vi "ConvertToAssociationType.vi"(0 "lineStyle":T3, 1 "EndArrowHead":T2, 2 "StartArrowHead":T2) -> (14 "RelationType":T1 items=["Depenency", "Inheritance", "Interface Implementation", "Association", "Aggregation", "Composite Aggregation"], 16 "Bi sirectional":bool)   [LabVIEW 2012, in "ClassRelationshipEdge.lvclass"]
uses:
  <resource>/Framework/Providers/Open_GDS/UML/ClassRelationshipEdge_class/ClassRelationshipEdge.lvclass
  <resource>/Framework/Providers/Open_GDS/UML/ArrowHead_class/ArrowHeadType.ctl
  <resource>/Framework/Providers/Open_GDS/UML/LineStyle_class/LineStyleType.ctl
  <resource>/Framework/Providers/Open_GDS/UML/ClassRelationshipEdge_class/private/AssociationType.ctl
  <resource>/Framework/Providers/Open_GDS/UML/ArrowHead_class/ArrowHead.lvclass
  <resource>/Framework/Providers/Open_GDS/UML/LineStyle_class/LineStyle.lvclass
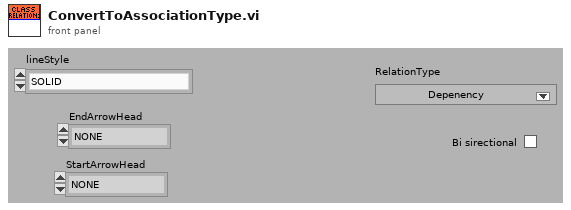
[diagram p1: front panel]
types:
  T1 = typedef "ClassRelationshipEdge.lvclass/AssociationType.ctl" = u16
  T2 = typedef "ArrowHead.lvclass/ArrowHeadType.ctl" = enum16{"NONE", "TRIANGLE", "BLACK_TRIANGLE", "V", "HALF_V", "DIAMOND", "BLACK_DIAMOND"}
  T3 = typedef "LineStyle.lvclass/LineStyleType.ctl" = enum16{"SOLID", "DOTTED"}
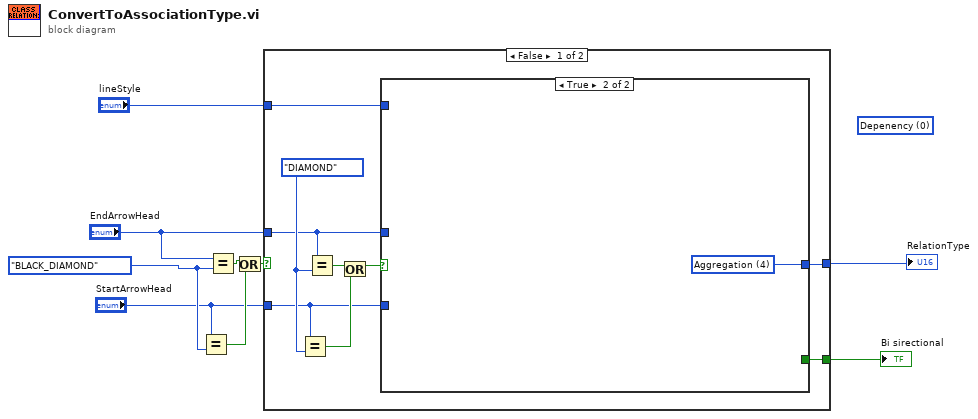
[diagram p0: block diagram]
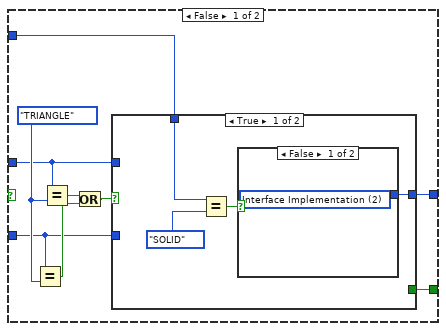
[diagram p2: hidden frame]
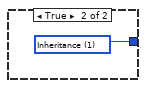
[diagram p3: hidden frame]
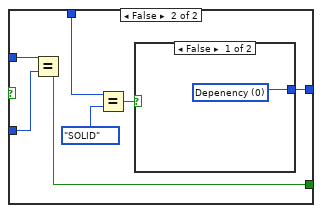
[diagram p4: hidden frame]
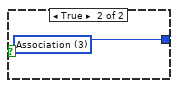
[diagram p5: hidden frame]
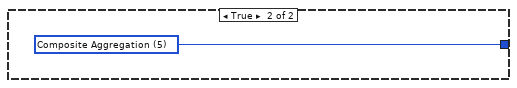
[diagram p6: hidden frame]
diagram:
  w7 = ArrowHeadType."BLACK_DIAMOND" ("y")
  (unwired) T1 0 items=["Depenency", "Inheritance", "Interface Implementation", "Association", "Aggregation", "Composite Aggregation"] ("RelationType")
  n1 = Equal?(x="StartArrowHead", y=w7) -> (x = y?=w5:bool)
  n2 = Equal?(x="EndArrowHead", y=w7) -> (x = y?=w9:bool)
  n3 = Or(x=w9, y=w5) -> (x .or. y?=w6:bool)
  n4 = case shown="False" w6 {
    tunnel: [w14 w44] -> w8
    tunnel: "StartArrowHead" -> [w12 _]
    tunnel: "EndArrowHead" -> [w13 _]
    tunnel: "lineStyle" -> [w11 _]
    tunnel: [w10 _] -> w1
    frame False {
      w16 = ArrowHeadType."DIAMOND" ("y")
      n5 = Equal?(x=w12, y=w16) -> (x = y?=w18:bool)
      n6 = Equal?(x=w13, y=w16) -> (x = y?=w17:bool)
      n7 = Or(x=w17, y=w18) -> (x .or. y?=w15:bool)
      n8 = case shown="True" w15 {
        tunnel: [w23 w43] -> w14
        tunnel: w13 -> [w21 _]
        tunnel: w12 -> [w20 _]
        tunnel: w11 -> [w22 _]
        tunnel: [w19 _] -> w10
        frame False {
          w27 = ArrowHeadType."TRIANGLE" ("y")
          n9 = Equal?(x=w20, y=w27) -> (x = y?=w25:bool)
          n10 = Equal?(x=w21, y=w27) -> (x = y?=w26:bool)
          n11 = Or(x=w26, y=w25) -> (x .or. y?=w24:bool)
          n12 = case shown="True" w24 {
            tunnel: [w31 w40] -> w23
            tunnel: w22 -> [w29 w38]
            tunnel: w21 -> [_ w37]
            tunnel: w20 -> [_ w36]
            tunnel: [_ w35] -> w19
            frame True {
              n13 = Equal?(x=w29, y=LineStyleType."SOLID" ("lineStyle")) -> (x = y?=w30:bool)
              n14 = case shown="False" w30 {
                tunnel: [w32 w33] -> w31
                frame False {
                  w32 = T1 2 items=["Depenency", "Inheritance", "Interface Implementation", "Association", "Aggregation", "Composite Aggregation"] ("RelationType")
                }
                frame True {
                  w33 = T1 1 items=["Depenency", "Inheritance", "Interface Implementation", "Association", "Aggregation", "Composite Aggregation"] ("RelationType")
                }
              }
            }
            frame False {
              n15 = Equal?(x=w37, y=w36) -> (x = y?=w35:bool)
              n16 = Equal?(x=w38, y=LineStyleType."SOLID" ("lineStyle")) -> (x = y?=w39:bool)
              n17 = case shown="False" w39 {
                tunnel: [w41 w42] -> w40
                frame False {
                  w41 = T1 0 items=["Depenency", "Inheritance", "Interface Implementation", "Association", "Aggregation", "Composite Aggregation"] ("RelationType")
                }
                frame True {
                  w42 = T1 3 items=["Depenency", "Inheritance", "Interface Implementation", "Association", "Aggregation", "Composite Aggregation"] ("RelationType")
                }
              }
            }
          }
        }
        frame True {
          w43 = T1 4 items=["Depenency", "Inheritance", "Interface Implementation", "Association", "Aggregation", "Composite Aggregation"] ("RelationType")
        }
      }
    }
    frame True {
      w44 = T1 5 items=["Depenency", "Inheritance", "Interface Implementation", "Association", "Aggregation", "Composite Aggregation"] ("RelationType")
    }
  }
  "RelationType" <- w8
  "Bi sirectional" <- w1
